vi "Launcher.vi"() -> ()   [LabVIEW 2021]
uses:
  OPC UA/OPC UA.lvclass
panel:
  in  "class path":path=path "C:/GitHub/OOP_OPC UA/PreUUT/PreUUT.lvclass"
  out "class name":string
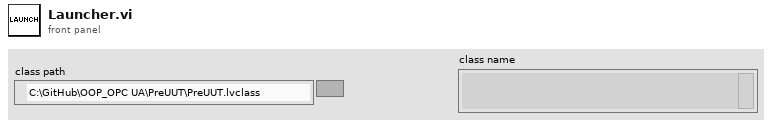
[diagram p1: front panel]
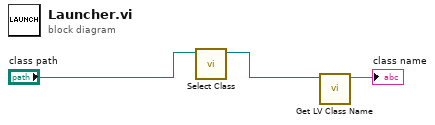
[diagram p0: block diagram]
diagram:
  n1 = call "Select Class.vi"("class path"="class path") -> ("Selected class reference"=w1:refnum<class "OPC UA.lvclass">)  [unwired: 9 in, 1 out]
  n2 = call <vilib>:"Get LV Class Name.vi"("object"=w1) -> ("class name"=→"class name":string)  [unwired: 9 in, 1 out]
